vi "Filter Wheel Initialize.vi"(8 "error in (no error)":errorcluster, 11 "Wheel Name":string="Default") -> (0 "error out":errorcluster, 2 "Filter Wheel Info":T1={"Num Wheels"=0, "Filters"=[], "Invalid Combinations"=[], "Addr"="", "Name"="", "Simulate"=FALSE, "Homing Parameters"={"Direction (F: CW)"=TRUE, "Speed"=150, "Accel"=400, "Min Distance"=2700, "Short Leg"=0, "Error Cnts"=0}, "Default Speed"=1000} {"Default Speed" min=20 max=4000 step=10}, 3 "Filter Wheel.lvclass":refnum<class "Filter Wheel.lvclass">)   [LabVIEW 2021]
uses:
  Filter Wheel Object/Filter Wheel.lvclass
  Filter Wheel configuration.ctl
  Filter Wheel Object/Filter Wheel Details.ctl
  Filter Wheel Arduino Control/Filter Wheel Arduino Homing cluster.ctl
  Filter Wheel Arduino Control/FW Arduino Control.lvclass
  C:/Development/prime/Prime-RIMAS/Filter Wheel/Filter Wheel Object/Filter Wheel.lvclass
  Filter Wheel Simulator/Filter Wheel Simulator.lvclass
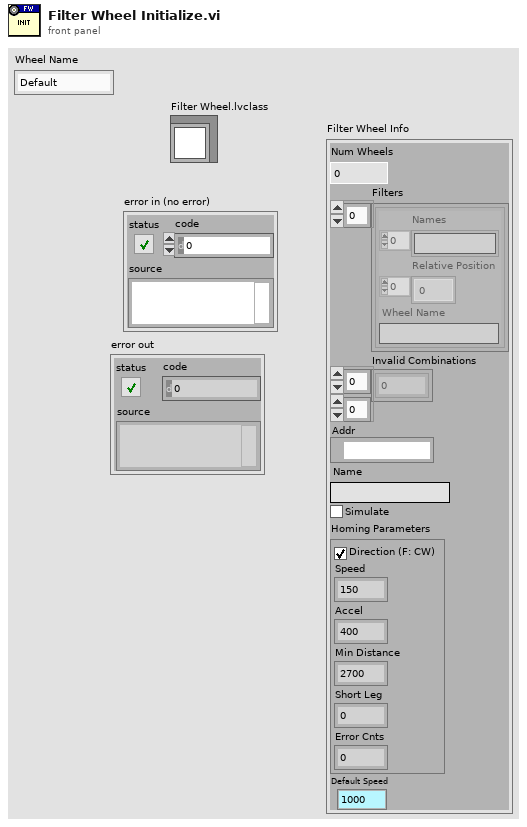
[diagram p1: front panel]
types:
  T1 = typedef "Filter Wheel.lvclass/Filter Wheel configuration.ctl" = cluster{"Num Wheels":i32, "Filters":T2[], "Invalid Combinations":i32[][], "Addr":refnum<visa-resource-name>, "Name":string, "Simulate":bool, "Homing Parameters":T3, "Default Speed":u16}
  T2 = typedef "Filter Wheel.lvclass/Filter Wheel Details.ctl" = cluster{"Names":string[], "Relative Position":i32[], "Wheel Name":string}
  T3 = typedef "Filter Wheel Arduino Homing cluster.ctl" = cluster{"Direction (F: CW)":bool, "Speed":i32, "Accel":i32, "Min Distance":i32, "Short Leg":i32, "Error Cnts":i32}
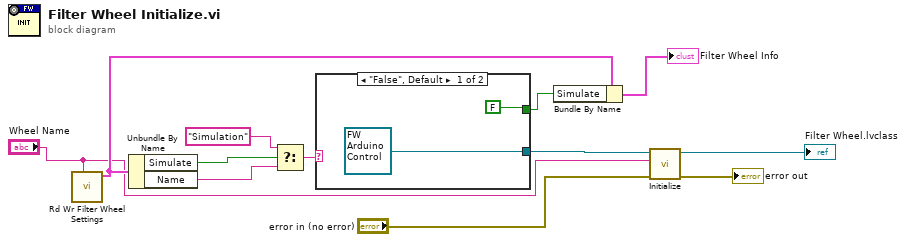
[diagram p0: block diagram]
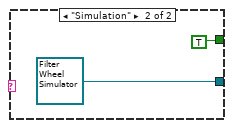
[diagram p2: hidden frame]
diagram:
  n1 = call "Rd Wr Filter Wheel Settings.vi"("Wheel Name"="Wheel Name") -> ("Filter Wheel Settings"=w4:T1)  [unwired: 9 in, 1 out]
  n2 = Unbundle By Name(w4) -> ("Simulate"=w11:bool, "Name"=w9:string)
  n3 = Select(t="Simulation" ("x"), s=w11, f=w9) -> (s? t:f=w8:string)
  n4 = case shown="\"False\", Default" w8 {
    tunnel: [refnum<class "FW Arduino Control.lvclass"> refnum ("FW Arduino Control.lvclass") refnum<class "Filter Wheel Simulator.lvclass"> refnum ("Filter Wheel Simulator.lvclass")] -> w7
    tunnel: [FALSE TRUE] -> w5
    frame "False", Default {
    }
    frame "Simulation" {
    }
  }
  n5 = Bundle By Name(cluster=w4, "Simulate"=w5) -> (→"Filter Wheel Info":T1)
  n6 = call-dynamic "Initialize.vi"("error in (no error)"="error in (no error)", "Name"="Wheel Name", "Filter Wheel in"=w7) -> ("error out"=→"error out":errorcluster, "Filter Wheel out"=→"Filter Wheel.lvclass":refnum<class "Filter Wheel.lvclass">)  [unwired: 7 in]
